vi "Start.vi"(7 "Table in":refnum<class "Table.lvclass">, 8 "error in":errorcluster) -> (0 "error out":errorcluster, 5 "Table out":refnum<class "Table.lvclass">)   [LabVIEW 2021, in "Table.lvclass"]
doc: "Assign chairs to Philosophers"
uses:
  Table.lvclass
  Philosopher/Philosopher.lvclass
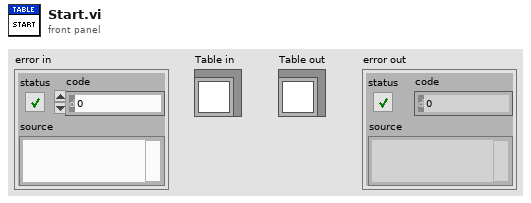
[diagram p1: front panel]
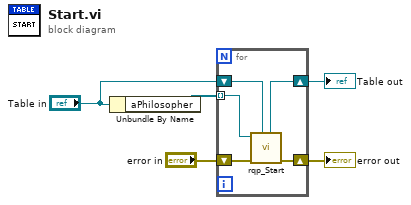
[diagram p0: block diagram]
diagram:
  n1 = Unbundle By Name("Table in") -> ("aPhilosopher"=w3:refnum<class "Philosopher.lvclass">[])
  n2 = for {
    tunnel: w3 -> [w8] mode=indexing
    shift-right: [w6] -> w1
    shift-left: "Table in" -> [w7]
    shift-right: [w9] -> w4
    shift-left: "error in" -> [w10]
    n3 = call "rqp_Start.vi"("Caller in"=w7, "error in"=w10, "Philosopher in"=w8) -> ("error out"=w9:errorcluster, "dup Caller out"=w6:refnum<class "Table.lvclass">)  [unwired: 6 in, 1 out]
  }
  "Table out" <- w1
  "error out" <- w4
